vi "Wait Ball CMD.vi"(10 "Delay ms":u32=500) -> ()   [LabVIEW 2014]
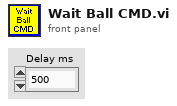
[diagram p1: front panel]
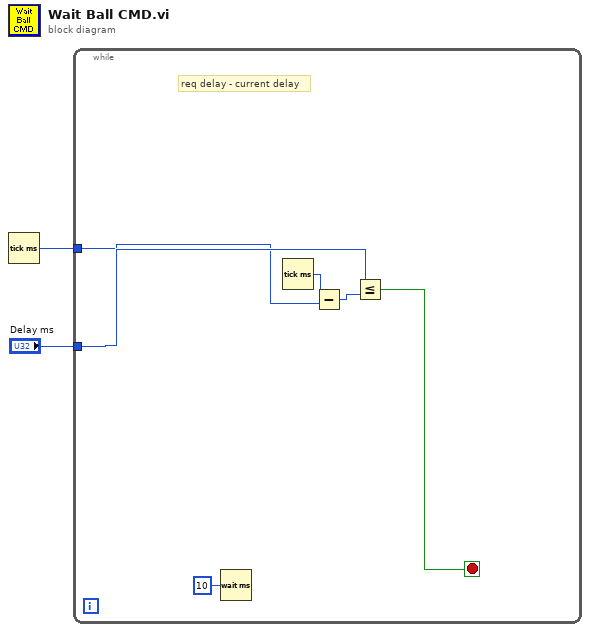
[diagram p0: block diagram]
diagram:
  n1 = Tick Count (ms)() -> (millisecond timer value=w1:u32)
  n2 = while {
    tunnel: "Delay ms" -> [w8]
    tunnel: w1 -> [w6]
    stop <- w7 stop-if-true
    # "req delay - current delay"
    n3 = Wait (ms)(milliseconds to wait=u32 10 ("millisecond multiple")) -> ()  [unwired: 1 out]
    n4 = Tick Count (ms)() -> (millisecond timer value=w3:u32)
    n5 = Subtract(x=w3, y=w6) -> (x-y=w4:u32)
    n6 = Less Or Equal?(x=w8, y=w4) -> (x <= y?=w7:bool)
  }
